vi "SetFirstMeasurementCycle.vi"() -> ()   [LabVIEW 2011]
panel:
  in  "FirstRoundMeasurement":bool
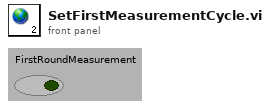
[diagram p1: front panel]
diagram:
